vi "Drive Chassies process.vi"(0 "error in":errorcluster) -> ()   [LabVIEW 2012]
uses:
  Drive Global Data.vi
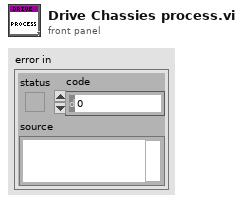
[diagram p1: front panel]
types:
  T1 = typedef "WPI_SolenoidValue.ctl" = enum16{"Off", "On", "Forward", "Reverse"}
  T2 = cluster{"Shifter?":bool, "Axisses":dbl[], "Shifter Value":T1}
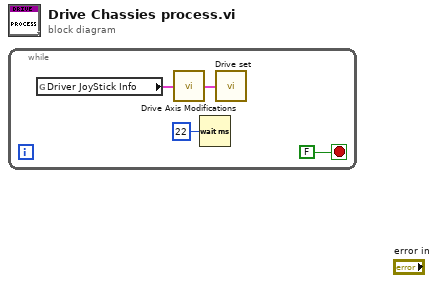
[diagram p0: block diagram]
diagram:
  n1 = while {
    stop <- FALSE stop-if-true
    n2 = global read "Drive Global Data.vi" "Driver JoyStick Info"() -> (w4:T2)
    n3 = call "Drive Axis Modifications.vi"("Driver JoyStick Info"=w4) -> ("Driver JoyStick Info 2"=w3:T2)
    n4 = Wait (ms)(milliseconds to wait=u32 22) -> ()  [unwired: 1 out]
    n5 = call "Drive set.vi"("Driver JoyStick Info"=w3) -> ()
  }
